vi "AudioTest.Tool - Convert Tab Delim Text to CSV.vi"() -> ()   [LabVIEW 2018]
panel:
  in  "Name":string
  out "error out":errorcluster
  in  "Dir":path=path "C:/MTE/Audio Test/Config/PlotLimits"
  in  "Text":string
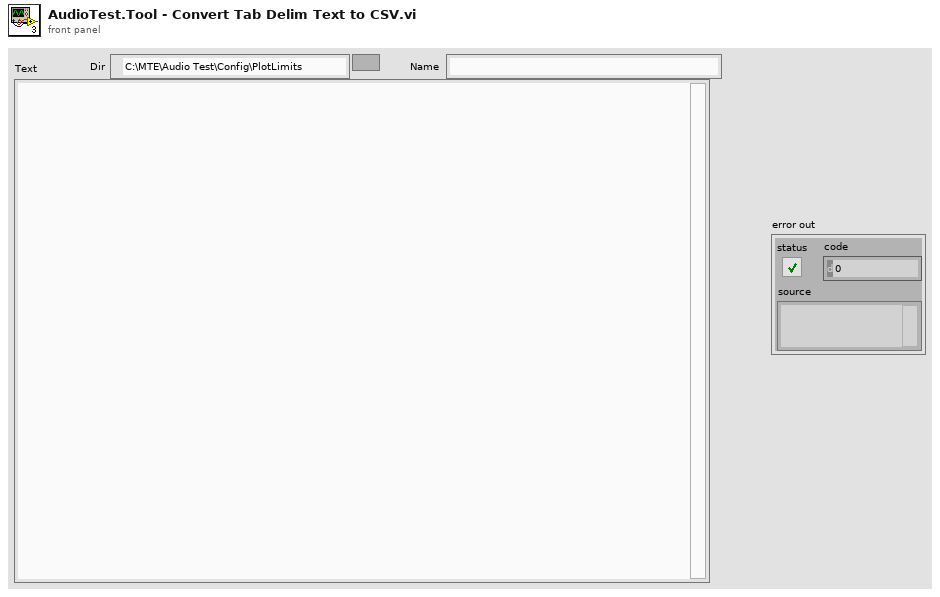
[diagram p1: front panel]
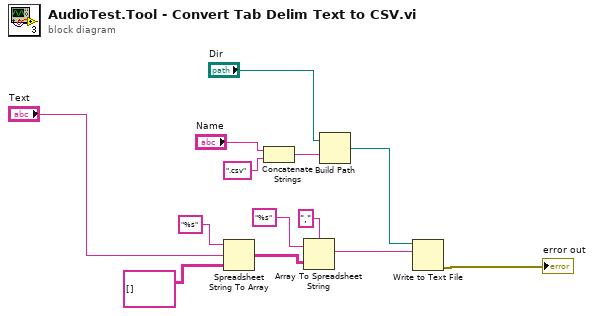
[diagram p0: block diagram]
diagram:
  n1 = Spreadsheet String To Array(format string="%s", spreadsheet string="Text", array type (2D Dbl)=string[][] []) -> (array=w9:string[][])  [unwired: 1 in]
  n2 = Concatenate Strings("Name", ".csv") -> (w3:string)
  n3 = Array To Spreadsheet String(delimiter (Tab)=",", array=w9, 3:"%s" ("format string")) -> (spreadsheet string=w7:string)
  n4 = Build Path(base path="Dir", name or relative path=w3) -> (appended path=w1:path)
  n5 = Write to Text File(file (use dialog)=w1, text=w7) -> (error out=→"error out":errorcluster)  [unwired: 2 in, 2 out]
